vi "serial_arduino_ABC.vi"() -> ()   [LabVIEW 2017]
uses:
  <vilib>/Instr/_visa.llb/VISA Configure Serial Port (Instr).vi
panel:
  out "String 2":string
  in  "stop":bool
  out "String":string
  out "Voltage":dbl
  out "Waveform Chart":dbl(graph)
  in  "flow control":u16(ring) items=["None"=0, "XON/XOFF"=1, "RTS/CTS"=2, "DTR/DSR"=4]
  in  "stop bits":u16(ring)=10 items=["1.0"=10, "1.5"=15, "2.0"=20]
  in  "parity":u16(ring) items=["None", "Odd", "Even", "Mark", "Space"]
  in  "data bits":u16=8 min=5 max=8 step=1
  in  "VISA resource name":refnum<visa-resource-name>="COM1"
  in  "baud rate":u32=9600
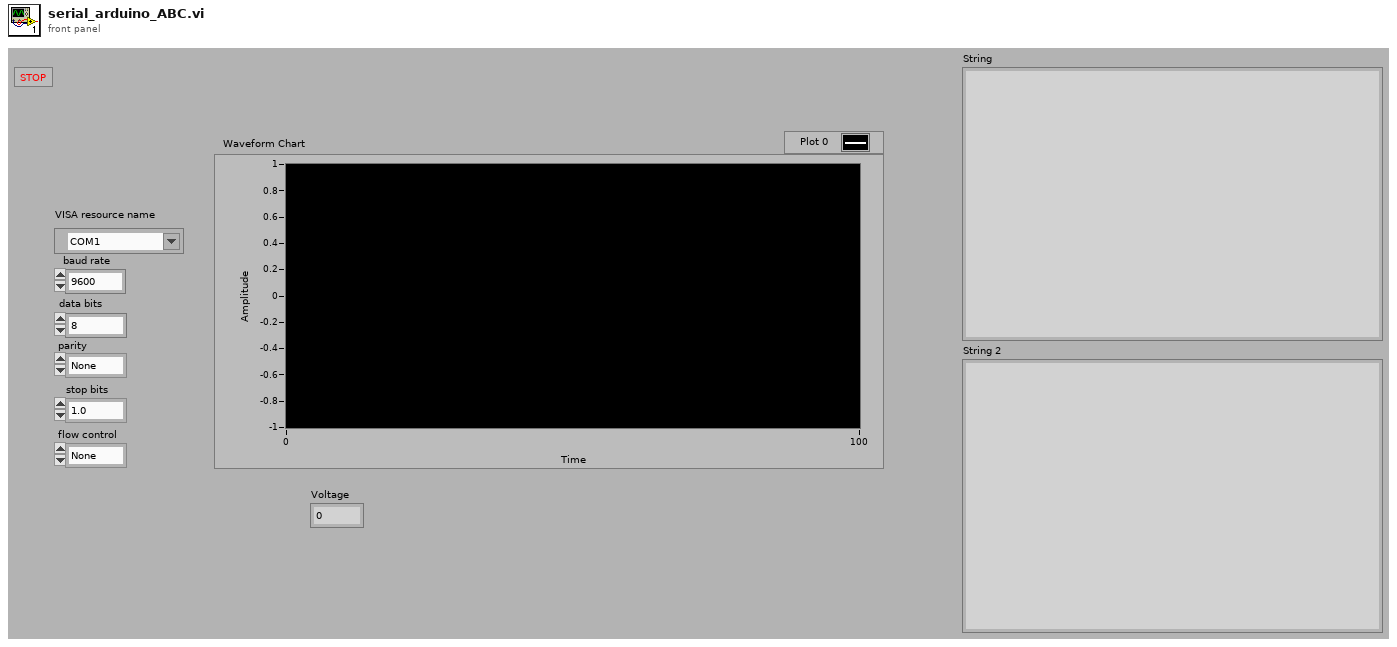
[diagram p1: front panel]
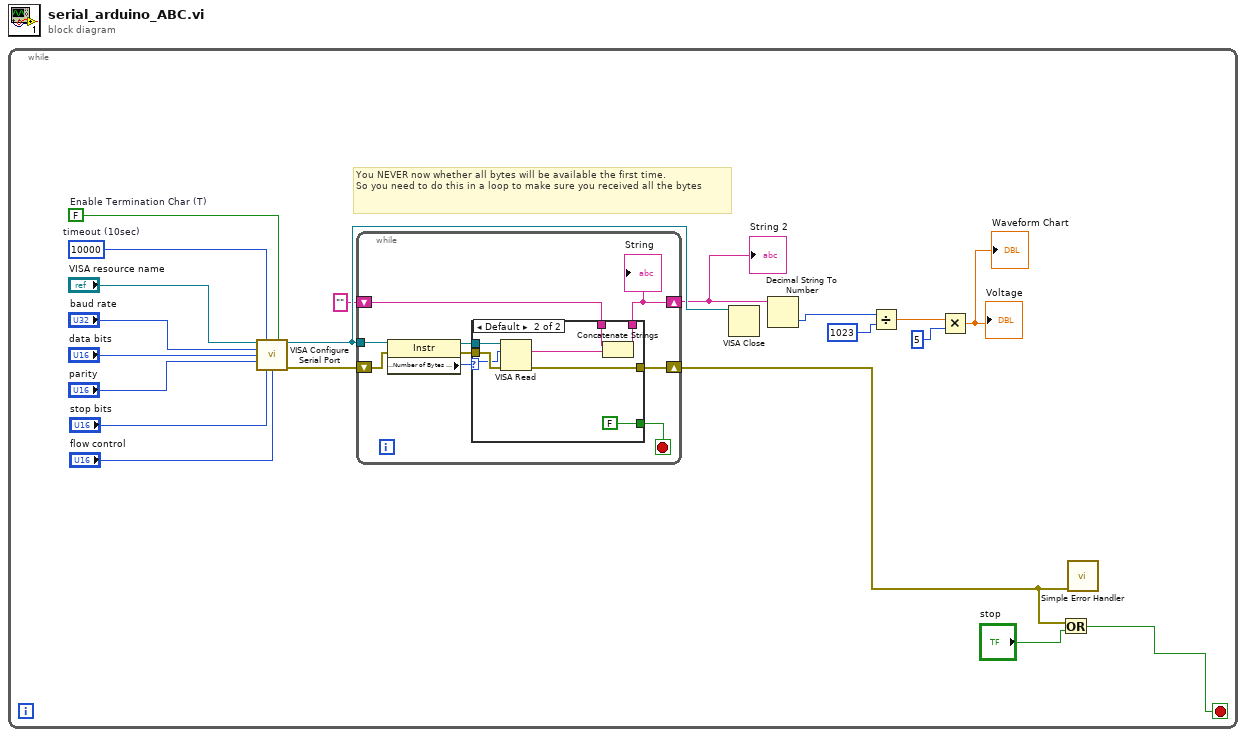
[diagram p0: block diagram]
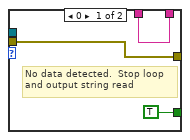
[diagram p2: hidden frame]
diagram:
  n1 = while {
    stop <- w1 stop-if-true
    w16 = FALSE  # Enable Termination Char (T)
    w17 = u32 10000  # timeout (10sec)
    # "You NEVER now whether all bytes will be available the first time.\nSo you need to do this in a loop to make sure you received all the bytes"
    n2 = call-poly "VISA Configure Serial Port"("VISA resource name"="VISA resource name", "timeout (10sec)"=w17, "Enable Termination\nChar (T)"=w16, "baud rate (9600)"="baud rate", "data bits (8)"="data bits", "parity (0:none)"="parity", "stop bits (10: 1 bit)"="stop bits", "flow control (0:none)"="flow control") -> ("VISA resource name out"=w11:refnum<visa-resource-name>, "error out"=w12:errorcluster)  [unwired: 1 in, 5 out]
    n3 = while {
      tunnel: w11 -> [w29]
      shift-right: [w25] -> w5
      shift-left: "" -> [w26]
      shift-right: [w22] -> w3
      shift-left: w12 -> [w21]
      stop <- w27 stop-if-true
      n4 = property class="Instr"(reference=w29, error in=w21) -> (reference out=w24:refnum<visa-resource-name>, error out=w23:errorcluster, "Serial Settings:Number of Bytes at Serial Port"=w28:u32)
      n5 = case shown="Default" w28 {
        selector: w28 -> [_ w34]
        tunnel: [TRUE FALSE] -> w27
        tunnel: w26 -> [w31 w38]
        tunnel: [w31 w39] -> w25
        tunnel: w24 -> [_ w40]
        tunnel: w23 -> [w30 w35]
        tunnel: [w30 w33] -> w22
        frame 0 {
          # "No data detected.  Stop loop\nand output string read"
        }
        frame Default {
          n6 = VISA Read(VISA resource name=w40, byte count=w34, error in (no error)=w35) -> (read buffer=w37:string, error out=w33:errorcluster)  [unwired: 2 out]
          n7 = Concatenate Strings(w38, w37) -> (w39:string)
        }
      }
      "String" <- w25
    }
    "String 2" <- w5
    n8 = VISA Close(VISA resource name=w11) -> ()  [unwired: 1 in, 1 out]
    n9 = Decimal String To Number(string=w5) -> (number=w10:i32)  [unwired: 1 in, 2 out]
    n10 = Divide(x=w10, y=1023) -> (x/y=w8:dbl)
    n11 = Multiply(x=w8, y=5) -> (x*y=→"Waveform Chart" →"Voltage":dbl)
    n12 = Or(x=w3, y="stop") -> (x .or. y?=w1:bool)
    n13 = call <vilib>:"Simple Error Handler.vi"("error in (no error)"=w3) -> ()  [unwired: 1 in, 8 out]
  }
